vi "getData.vi"(11 "Local Debug":bool) -> ()   [LabVIEW 2016]
uses:
  <vilib>/httpClient/LabVIEWHTTPClient.lvlib
  msg7171_linux.llb/send single message.vi
  msg7171_linux.llb/send multiple messages.vi
  <vilib>/httpClient/ClientHandle.ctl
panel:
  in  "exit":bool
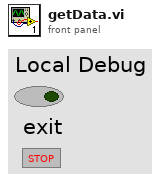
[diagram p1: front panel]
types:
  T1 = typedef "LabVIEWHTTPClient.lvlib/ClientHandle.ctl" = refnum<k1>
  T2 = cluster{"go":bool, "Http session":T1, "URL prefex":string}
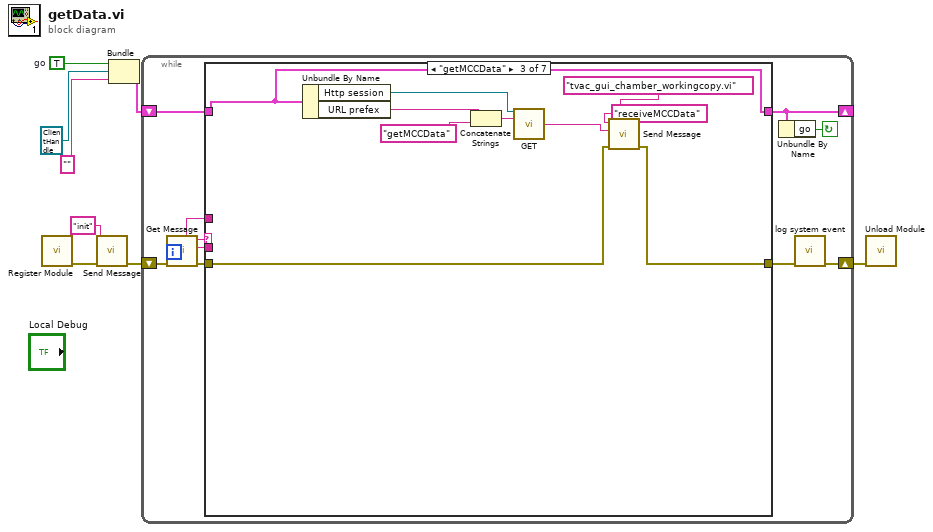
[diagram p0: block diagram]
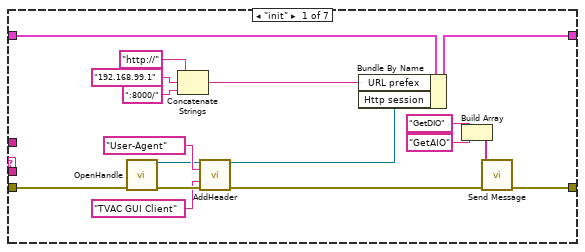
[diagram p2: hidden frame]
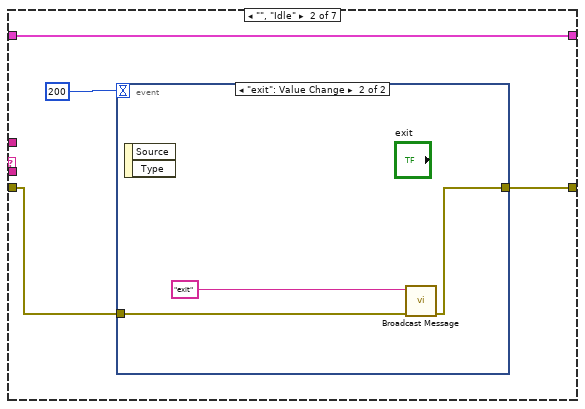
[diagram p3: hidden frame]
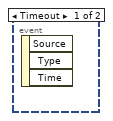
[diagram p4: hidden frame]
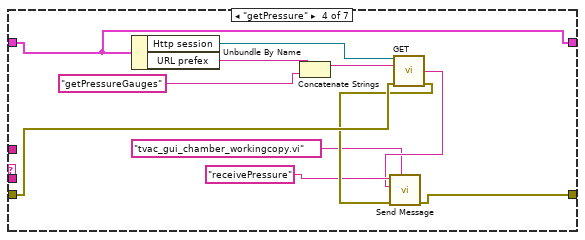
[diagram p5: hidden frame]
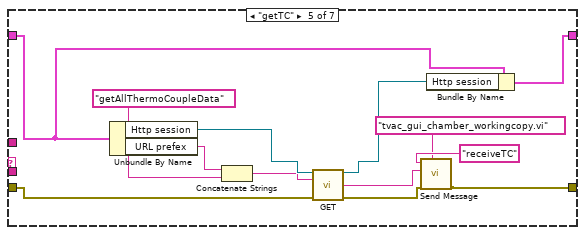
[diagram p6: hidden frame]
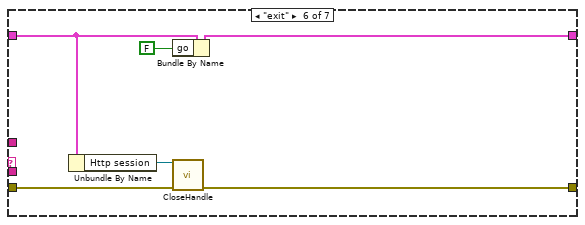
[diagram p7: hidden frame]
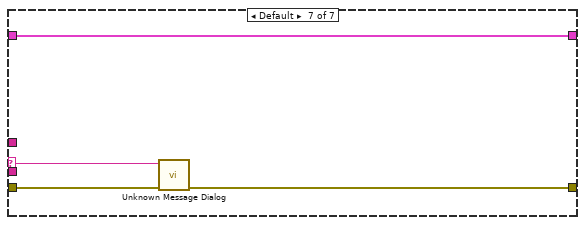
[diagram p8: hidden frame]
diagram:
  w6 = TRUE  # go
  n1 = call "Register Module.vi"() -> ("error out"=w2:errorcluster)  [unwired: 10 in, 1 out]
  n2 = call-poly "Send Message.vi"("error in (no error)"=w2, "event"="init") -> ("error out"=w1:errorcluster)  [unwired: 9 in]
  n3 = Bundle("go"=w6, "Http session"=T1 refnum, "URL prefex"="") -> (w8:T2)  [unwired: 1 in]
  n4 = while {
    shift-left: w8 -> [w15]
    shift-right: [w13] -> _
    shift-right: [w11] -> w7
    shift-left: w1 -> [w18]
    stop <- w12 continue-if-true
    n5 = call "Get Message.vi"("error in (no error)"=w18) -> ("error out"=w16:errorcluster, "event buffer"=w17:string, "event"=w14:string, "source"=w9:string)  [unwired: 7 in]
    n6 = case shown="\"getMCCData\"" w14 {
      selector: w14 -> [_ _ _ _ _ _ w84]
      tunnel: [w26 w37 w43 w53 w70 w82 w86] -> w13
      tunnel: w15 -> [w35 w37 w43 w53 w72 w77 w86]
      tunnel: w17 -> [_ _ _ _ _ _ _]
      tunnel: w16 -> [w30 w39 w45 w59 w73 w80 w85]
      tunnel: [w22 w38 w44 w57 w68 w79 w83] -> w10
      tunnel: w9 -> [_ _ _ _ _ _ _]
      frame "init" {
        n7 = call <vilib>:"OpenHandle.vi"("error in (no error)"=w30) -> ("client handle out"=w31:T1, "error out"=w34:errorcluster)  [unwired: 13 in]
        n8 = Concatenate Strings("http://" ("url"), "192.168.99.1" ("Address"), ":8000/" ("url")) -> (w25:string)
        n9 = call <vilib>:"AddHeader.vi"("client handle"=w31, "header"="User-Agent", "value"="TVAC GUI Client", "error in (no error)"=w34) -> ("client handle out"=w24:T1, "error out"=w23:errorcluster)  [unwired: 10 in]
        n10 = Bundle By Name(cluster=w35, "URL prefex"=w25, "Http session"=w24) -> (w26:T2)
        n11 = Build Array("GetDIO" ("event"), "GetAIO" ("event")) -> (w20:string[])
        n12 = call-poly "Send Message.vi"("error in (no error)"=w23, "event"=w20) -> ("error out"=w22:errorcluster)  [unwired: 9 in]
      }
      frame "", "Idle" {
        n13 = event shown="[1] \"exit\": Value Change" {
          selector: _ -> [_ _]
          dyn-events: _ -> [_ _]
          timeout: 200 ("Numeric") -> [_ _]
          tunnel: w39 -> [_ w41]
          tunnel: [_ w40] -> w38
          event Timeout {
            n14 = event-data() -> ()  [unwired: 1 in, 3 out]
          }
          event "exit": Value Change {
            n15 = event-data() -> ()  [unwired: 1 in, 2 out]
            n16 = call "Broadcast Message.vi"("error in (no error)"=w41, "event"="exit") -> ("error out"=w40:errorcluster)  [unwired: 9 in]
          }
        }
      }
      frame "getMCCData" {
        n17 = Unbundle By Name(w43) -> ("Http session"=w49:T1, "URL prefex"=w51:string)
        n18 = Concatenate Strings(w51, "getMCCData" ("url")) -> (w52:string)
        n19 = call <vilib>:"GET.vi"("client handle"=w49, "url"=w52) -> ("body"=w47:string)  [unwired: 10 in, 3 out]
        n20 = call-poly "Send Message.vi"("Destination Module"="tvac_gui_chamber_workingcopy.vi", "error in (no error)"=w45, "event buffer"=w47, "event"="receiveMCCData" ("url")) -> ("error out"=w44:errorcluster)  [unwired: 7 in]
      }
      frame "getPressure" {
        n21 = Unbundle By Name(w53) -> ("Http session"=w60:T1, "URL prefex"=w62:string)
        n22 = Concatenate Strings(w62, "getPressureGauges" ("url")) -> (w63:string)
        n23 = call <vilib>:"GET.vi"("client handle"=w60, "url"=w63, "error in (no error)"=w59) -> ("body"=w55:string, "error out"=w58:errorcluster)  [unwired: 9 in, 2 out]
        n24 = call-poly "Send Message.vi"("Destination Module"="tvac_gui_chamber_workingcopy.vi", "error in (no error)"=w58, "event buffer"=w55, "event"="receivePressure" ("url")) -> ("error out"=w57:errorcluster)  [unwired: 7 in]
      }
      frame "getTC" {
        n25 = Unbundle By Name(w72) -> ("Http session"=w76:T1, "URL prefex"=w64:string)
        n26 = Concatenate Strings(w64, "getAllThermoCoupleData" ("url")) -> (w75:string)
        n27 = call <vilib>:"GET.vi"("client handle"=w76, "url"=w75, "error in (no error)"=w73) -> ("client handle out"=w71:T1, "body"=w66:string, "error out"=w69:errorcluster)  [unwired: 9 in, 1 out]
        n28 = call-poly "Send Message.vi"("Destination Module"="tvac_gui_chamber_workingcopy.vi", "error in (no error)"=w69, "event buffer"=w66, "event"="receiveTC" ("url")) -> ("error out"=w68:errorcluster)  [unwired: 7 in]
        n29 = Bundle By Name(cluster=w72, "Http session"=w71) -> (w70:T2)
      }
      frame "exit" {
        n30 = Unbundle By Name(w77) -> ("Http session"=w78:T1)
        n31 = Bundle By Name(cluster=w77, "go"=FALSE ("Bundle Element")) -> (w82:T2)
        n32 = call <vilib>:"CloseHandle.vi"("client handle"=w78, "error in (no error)"=w80) -> ("error out"=w79:errorcluster)  [unwired: 13 in]
      }
      frame Default {
        n33 = call "Unknown Message Dialog.vi"("error in (no error)"=w85, "event name"=w84) -> ("error out"=w83:errorcluster)  [unwired: 9 in]
      }
    }
    n34 = Unbundle By Name(w13) -> ("go"=w12:bool)
    n35 = call "log system event.vi"("error in (no error)"=w10) -> ("error out"=w11:errorcluster)  [unwired: 9 in, 1 out]
  }
  n36 = call "Unload Module.vi"("error in (no error)"=w7) -> ()  [unwired: 10 in, 1 out]
